vi "Deactivate Subscription Policy.vi"(8 "error in (no error)":errorcluster, 11 "Subscription Policy":T1) -> (0 "error out":errorcluster)   [LabVIEW 2018, in "MVA Framework.lvlib" / "IMediator.lvlib" / "ISubscriptionPolicy.lvclass"]
doc: "停用订阅策略"
uses:
  ISubscriptionPolicy.lvclass
  ISubscriptionPolicy Reference.ctl
panel:
  out "Subscription Policy Out":T1
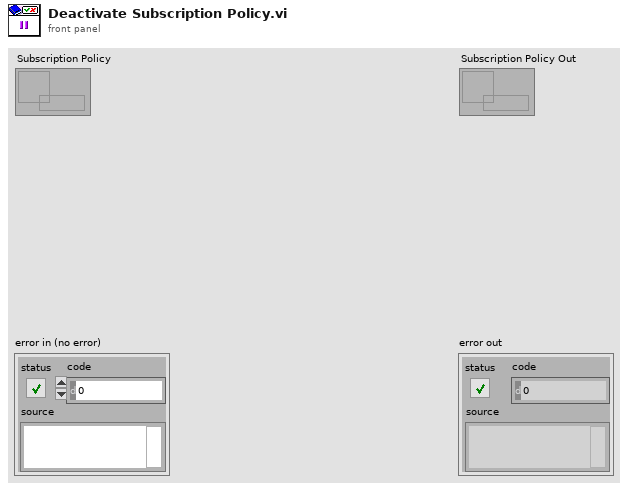
[diagram p1: front panel]
types:
  T1 = typedef "MVA Framework.lvlib/IMediator.lvlib/ISubscriptionPolicy.lvclass/ISubscriptionPolicy Reference.ctl" = refnum<data-value>
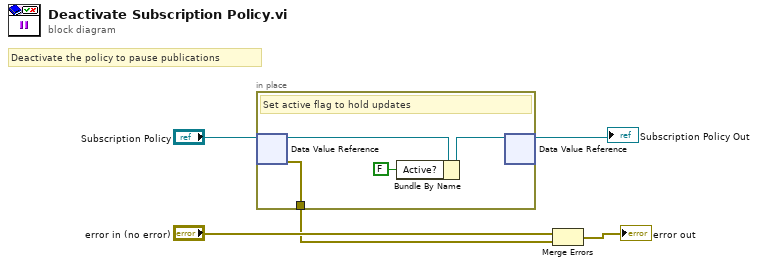
[diagram p0: block diagram]
diagram:
  # "Deactivate the policy to pause publications"
  n1 = in-place {
    in-place-border: [w8] -> w2
    # "Set active flag to hold updates"
    n2 = in-place-dvr #1("Subscription Policy") -> (w9:refnum<class "ISubscriptionPolicy.lvclass">, w8:errorcluster)
    n3 = Bundle By Name(cluster=w9, "Active?"=FALSE) -> (w7:refnum<class "ISubscriptionPolicy.lvclass">)
    n4 = in-place-dvr #1(w7) -> (→"Subscription Policy Out":T1)  [unwired: 1 out]
  }
  n5 = Merge Errors("error in (no error)", w2) -> (→"error out":errorcluster)
